vi "Top Level.vi"() -> ()   [LabVIEW 2017]
uses:
  <vilib>/rvi/Emulation/niFpgaGetClockAttributes.vi
  <vilib>/rvi/Emulation/niFpgaSctlEmulationGetInTimedLoop.vi
  <vilib>/rvi/Emulation/niFpgaEmulationReportErrorSimple.vi
  <vilib>/rvi/interface/RandomDataEmulation/niFpgaRandomDataHandleErrors.vi
  <vilib>/rvi/eio/common/nirviEmuTemplateMethod_errors.vi
  <vilib>/rvi/Emulation/niFpgaCriticalErrorInLSC.vi
  <vilib>/rvi/DataTransferAndStorage/Container/XNode/niFpgaContainer.xnode
  <vilib>/rvi/interface/RandomDataEmulation/nirviRandomDataFpgaReadWriteTemplate.vi
  <vilib>/eio/EIONode/EIONode.xnode
panel:
  out "Z AO":i16
  in  "Z Signal Amplitude":u16=32768
  in  "Z Accumulator Increment":u32=100000
  out "Z Accumulator Value":u32 format="%.3e"
  in  "Z Phase Shift":u32
  out "AO DMA Overflow":bool
  out "X AO":i16
  in  "Reset Accumulator":bool
  out "Actual Gen Rate (ticks)":u32
  in  "X Signal Amplitude":u16=32768
  in  "Update Rate (ticks)":u32=40
  in  "X Accumulator Increment":u32=100000
  out "X Accumulator Value":u32 format="%.3e"
  in  "X Phase Shift":u32
  in  "Stop":bool
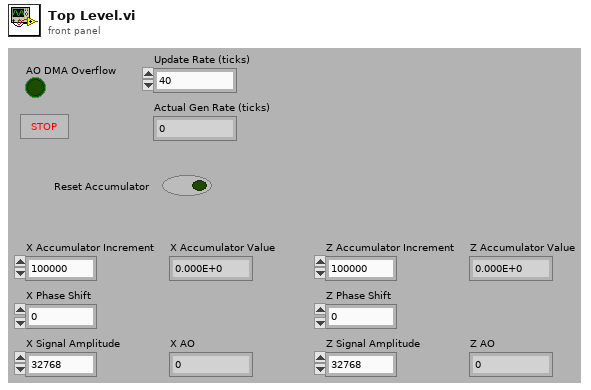
[diagram p1: front panel]
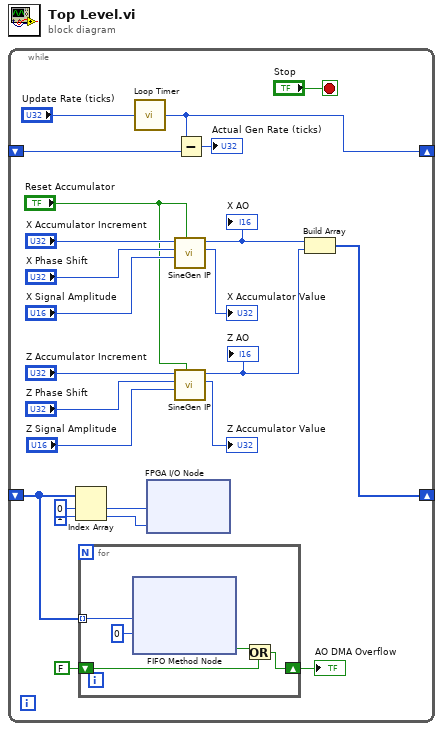
[diagram p0: block diagram]
diagram:
  n1 = while {
    shift-right: [w10] -> _
    shift-left: _ -> [w6]
    shift-right: [w21] -> _
    shift-left: _ -> [w22]
    stop <- "Stop" stop-if-true
    n2 = Index Array(array=w6, index #1=0 ("index"), index #2=1 ("index")) -> (element #1=w8:i16, element #2=w7:i16)
    n3 = for {
      tunnel: w6 -> [w28] mode=indexing
      shift-right: [w27] -> w4
      shift-left: FALSE -> [w26]
      n4 = xnode ("FIFO Method Node")("Element"=w28, "Timeout"=0) -> ("Timed Out?"=w25:bool)  [unwired: 1 in, 1 out]
      n5 = Or(x=w25, y=w26) -> (x .or. y?=w27:bool)
    }
    "AO DMA Overflow" <- w4
    n6 = call "Loop Timer"("Count(Ticks)"="Update Rate (ticks)") -> ("Tick Count(Ticks)"=w21:u32)
    n7 = xnode "FPGA I/O Node"("X Galvo"=w8, "Z Galvo"=w7) -> ()  [unwired: 2 in, 2 out]
    n8 = call "SineGen IP.vi"("Reset Accumulator"="Reset Accumulator", "Signal Amplitude (x 2^15)"="X Signal Amplitude", "Phase Shift"="X Phase Shift", "Accumulator Increment"="X Accumulator Increment") -> ("Accumulator Value"=→"X Accumulator Value":u32, "Signal Value"=w12:i16)  [unwired: 6 in]
    "X AO" <- w12
    n9 = call "SineGen IP.vi"("Reset Accumulator"="Reset Accumulator", "Signal Amplitude (x 2^15)"="Z Signal Amplitude", "Phase Shift"="Z Phase Shift", "Accumulator Increment"="Z Accumulator Increment") -> ("Accumulator Value"=→"Z Accumulator Value":u32, "Signal Value"=w11:i16)  [unwired: 6 in]
    "Z AO" <- w11
    n10 = Subtract(x=w21, y=w22) -> (x-y=→"Actual Gen Rate (ticks)":u32)
    n11 = Build Array(w12, w11) -> (w10:i16[])
  }
